vi "AB_820_850_ConvertProtoForPrevious.vi"(8 "error in (no error)":errorcluster, 10 "Path":path, 11 "dataSource in":cluster{"vipInfo":T1}) -> (0 "error out":errorcluster, 3 "dataSource out":cluster{"vipInfo":T1})   [LabVIEW 2020]
doc: "Reads and writes the data to the object property bag."
uses:
  <vilib>/AppBuilder/ABAPI Dist VI Proto Info.ctl
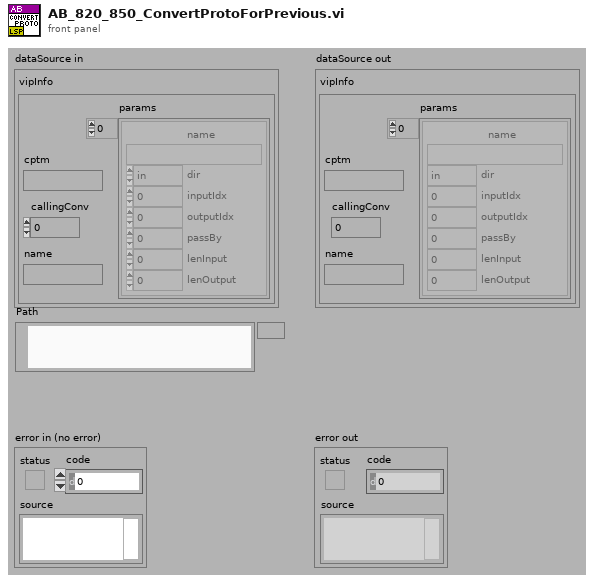
[diagram p1: front panel]
types:
  T1 = typedef "ABAPI Dist VI Proto Info.ctl" = cluster{"cptm":string, "params":cluster{"name":string, "dir":enum32{"in", "out", "in/out", "length"}, "inputIdx":i32, "outputIdx":i32, "passBy":i32, "lenInput":i32, "lenOutput":i32}[], "callingConv":i32, "name":string}
  T2 = cluster{"cptm":string, "params":cluster{"name":string, "dir":enum32{"in", "out", "in/out", "length"}, "inputIdx":i32, "outputIdx":i32, "passBy":i32, "lenInput":i32, "lenOutput":i32}[], "callingConv":i32, "name":string}
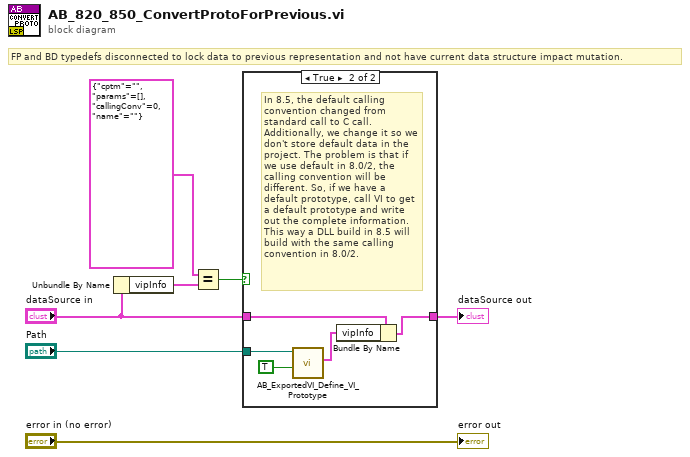
[diagram p0: block diagram]
diagram:
  # "FP and BD typedefs disconnected to lock data to previous representation and not have current data structure impact mutation."
  n1 = Unbundle By Name("dataSource in") -> ("vipInfo"=w6:T1)
  n2 = Equal?(x=T2 {"cptm"="", "params"=[], "callingConv"=0, "name"=""} ("vipInfo"), y=w6) -> (x = y?=w4:bool)
  n3 = case shown="True" w4 {
    tunnel: "Path" -> [_ w13]
    tunnel: "dataSource in" -> [w8 w11]
    tunnel: [w8 w9] -> w1
    frame False {
    }
    frame True {
      # "In 8.5, the default calling convention changed from standard call to C call. Additionally, we change it so we don't store default data in the project. The problem is that if we use default in 8.0/2, the calling convention will be different. So, if we have a default prototype, call VI to get a default prototype and write out the complete information. This way a DLL build in 8.5 will build with the same calling convention in 8.0/2."
      n4 = call <vilib>:"AB_ExportedVI_Define_VI_Prototype.vi"("verify only"=TRUE, "path"=w13) -> ("vipInfo out"=w10:T1)  [unwired: 7 in, 2 out]
      n5 = Bundle By Name(cluster=w11, "vipInfo"=w10) -> (w9:cluster{"vipInfo":T1})
    }
  }
  "dataSource out" <- w1
  "error out" <- "error in (no error)"
